vi "testUnflattenLengthFromXML.vi"() -> ()   [LabVIEW 2012, in "UnitsAndXML.lvlib"]
uses:
  <userlib>/Common/UnitsAndXML/UnitsAndXML.lvlib
  <userlib>/Common/UnitsAndXML/FlattenItemWithUnitToXML/FlattenLengthToXML/LengthUnit.ctl
  <userlib>/Common/UnitsAndXML/UnflattenItemWithUnitFromXML/UnflattenLengthFromXML/typeMethods/unflattenLengthFromXML_Array.vi
  <userlib>/Common/UnitsAndXML/UnflattenItemWithUnitFromXML/UnflattenLengthFromXML/typeMethods/unflattenLengthFromXML_Scalar.vi
panel:
  out "error out":errorcluster
  out "length":dbl[unit][](array[numeric])
  out "length":dbl[unit]
  in  "lengthUnitInXML":T1
  in  "xmlStringArray":string="<length>15</length>\r\n<length>30</length>\r\n<length>45</length>\r\n<length>60</length>"
  in  "xmlStringScalar":string="<length>15</length>"
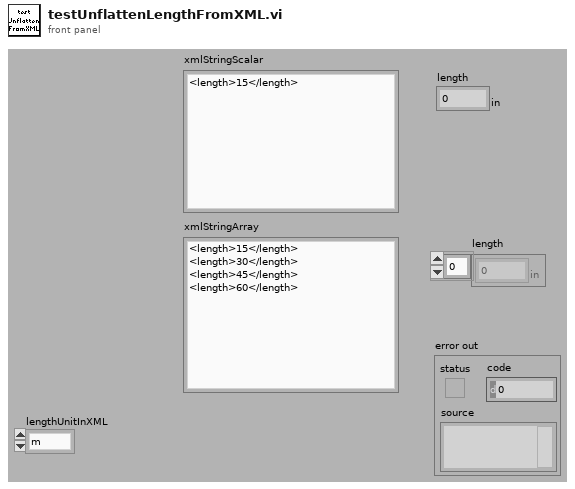
[diagram p1: front panel]
types:
  T1 = typedef "UnitsAndXML.lvlib/LengthUnit.ctl" = enum16{"m", "Angstrom", "AU", "chain", "cm", "cubit", "fathom", "fermi", "ft", "furlong", "hubble", "in", "ly", "mi", "mm", "rod", "um", "yd"}
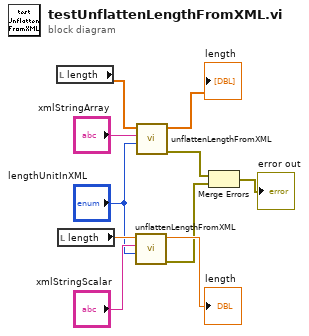
[diagram p0: block diagram]
diagram:
  n1 = local read "length"() -> (w3:dbl[unit][])
  n2 = local read "length"() -> (w9:dbl[unit])
  n3 = call-poly <userlib>:"unflattenLengthFromXML.vi"("lengthUnitInXML"="lengthUnitInXML", "xmlString"="xmlStringScalar", "lengthForType"=w9) -> ("error out"=w5:errorcluster, "length"=→"length":dbl[unit])  [unwired: 7 in]
  n4 = call-poly <userlib>:"unflattenLengthFromXML.vi"("lengthUnitInXML"="lengthUnitInXML", "xmlString"="xmlStringArray", "lengthForType"=w3) -> ("error out"=w6:errorcluster, "length"=→"length":dbl[unit][])  [unwired: 7 in]
  n5 = Merge Errors(w6, w5) -> (→"error out":errorcluster)
